vi "Simple_Frequency_Reader.vi"() -> ()   [LabVIEW 2013]
uses:
  <vilib>/S3DK/PMU Recorder Light/PMU Recorder Light.lvlib
panel:
  in  "Quit":bool
  out "Waveform Chart":waveform(sgl)[](graph)
  in  "Refresh Rate":i64(ring)=200 items=["50 Hz"=20, "20 Hz"=50, "10 Hz"=100, "5 Hz"=200, "2 Hz"=500, "1 Hz"=1000, "Every 2 sec"=2000, "Every 5 sec"=5000, "Every 10 sec"=10000, "Every minute"=60000]
  in  "error in (no error)":errorcluster
  out "error out":errorcluster
  # "INPUT"
  # "INTERMEDIATE"
  # "OUTPUT"
  # "USAGE:  Press play. The VI will start the PRL itself and wait for the connection to be established.\n(you will still need to configure the PRL first. If the Simple Frequency Reader works, then this works)"
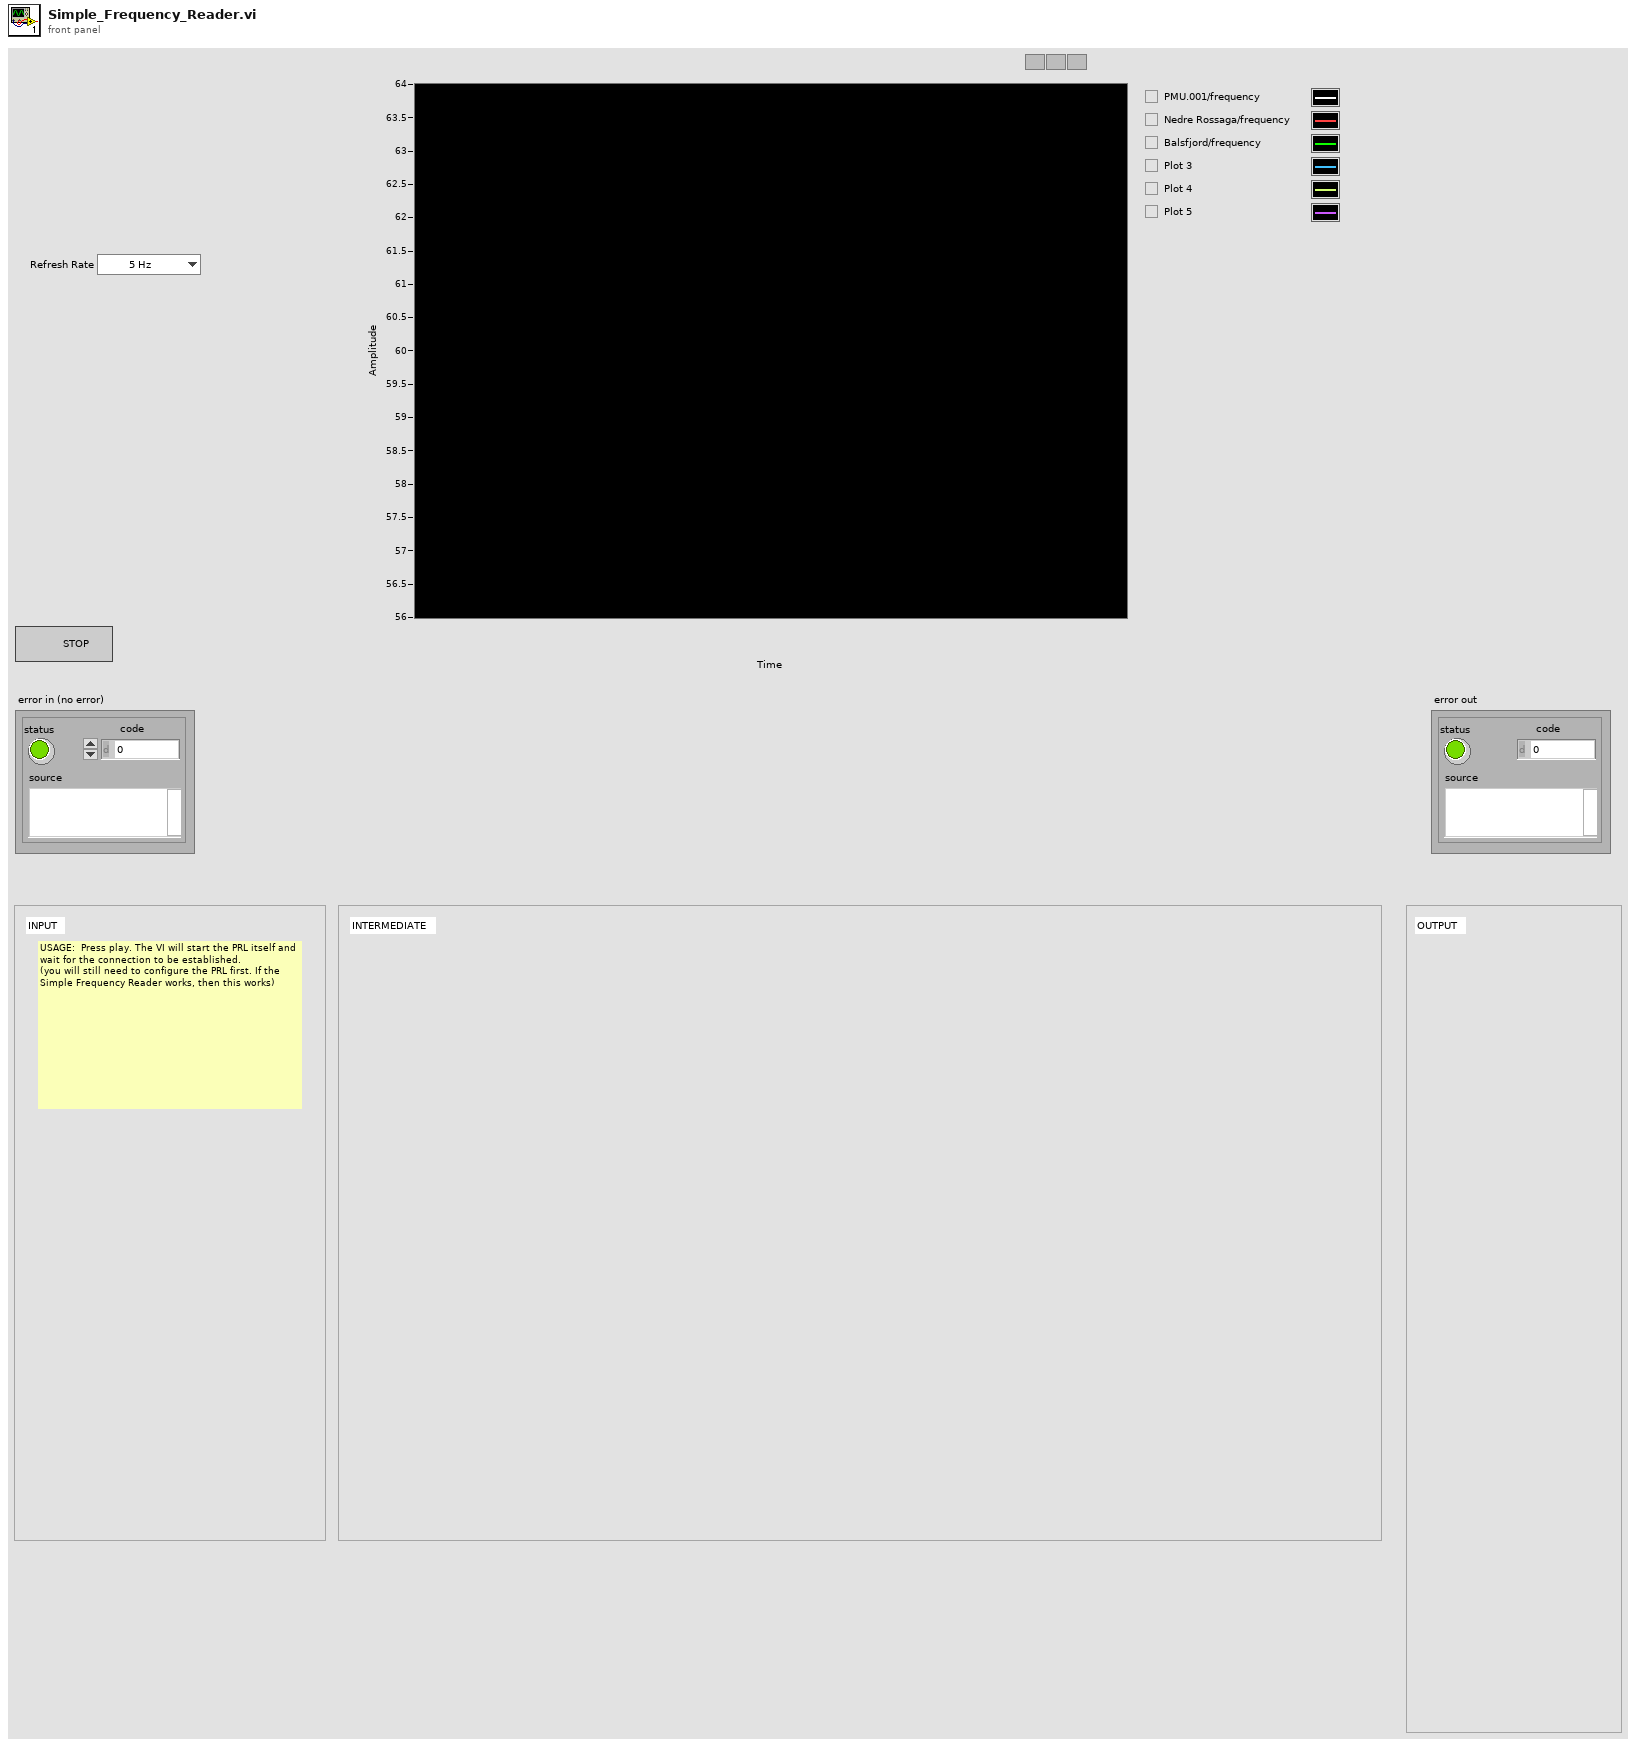
[diagram p1: front panel]
types:
  T1 = enum16{"Run", "Startup", "Get Status", "Pause", "Continue", "Shutdown", "Abort", "Open Panel", "Close Panel"}
  T2 = enum16{"Filter Signals", "Get All Signal Names", "Select Signals on Name", "Select Frequency Only", "Get Selected Signal Names"}
  T3 = cluster{"Phasor":string[], "Analog":string[], "Digital":string[]}
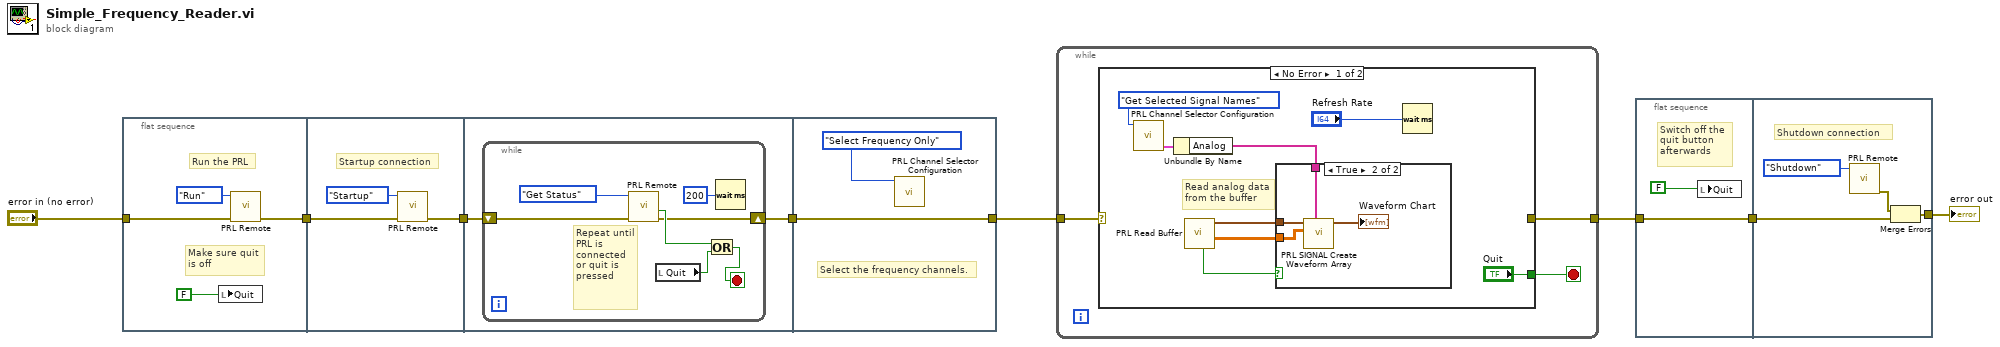
[diagram p0: block diagram]
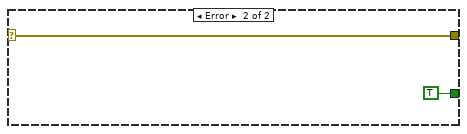
[diagram p3: hidden frame]
diagram:
  n1 = flat-sequence {
    tunnel: "error in (no error)" -> [w10]
    tunnel: [w9] -> w8
    tunnel: w8 -> [w14]
    tunnel: [w13] -> w7
    tunnel: w7 -> [w17]
    tunnel: [w16] -> w6
    tunnel: w6 -> [w25]
    tunnel: [w25] -> w2
    frame #0 {
      # "Make sure quit\nis off"
      # "Run the PRL"
      n2 = local write "Quit"(FALSE ("Quit")) -> ()
      n3 = call <vilib>:"PRL Remote.vi"("error in (no error)"=w10, "Action"=T1."Run") -> ("error out"=w9:errorcluster)  [unwired: 4 in, 5 out]
    }
    frame #1 {
      # "Startup connection"
      n4 = call <vilib>:"PRL Remote.vi"("error in (no error)"=w14, "Action"=T1."Startup") -> ("error out"=w13:errorcluster)  [unwired: 4 in, 5 out]
    }
    frame #2 {
      n5 = while {
        shift-right: [w18] -> w16
        shift-left: w17 -> [w19]
        stop <- w22 stop-if-true
        # "Repeat until PRL is connected or quit is pressed"
        n6 = call <vilib>:"PRL Remote.vi"("error in (no error)"=w19, "Action"=T1."Get Status") -> ("error out"=w18:errorcluster, "Connected"=w20:bool)  [unwired: 4 in, 4 out]
        n7 = local read "Quit"() -> (w21:bool)
        n8 = Or(x=w20, y=w21) -> (x .or. y?=w22:bool)
        n9 = Wait (ms)(milliseconds to wait=u32 200) -> ()  [unwired: 1 out]
      }
    }
    frame #3 {
      # "Select the frequency channels."
      n10 = call <vilib>:"PRL Channel Selector Configuration.vi"("Action"=T2."Select Frequency Only") -> ()  [unwired: 10 in, 1 out]
    }
  }
  n11 = while {
    tunnel: w2 -> [w28]
    tunnel: [w27] -> w3
    stop <- w29 stop-if-true
    n12 = case shown="No Error" w28 {
      selector: w28 -> [_ w43]
      tunnel: ["Quit" TRUE] -> w29
      tunnel: [_ w43] -> w27
      frame No Error {
        # "Read analog data\nfrom the buffer"
        n13 = call <vilib>:"PRL Channel Selector Configuration.vi"("Action"=T2."Get Selected Signal Names") -> ("Signal Names Out"=w35:T3)  [unwired: 10 in]
        n14 = Unbundle By Name(w35) -> ("Analog"=w34:string[])
        n15 = call <vilib>:"PRL Read Buffer .vi"() -> ("Analog Signals"=w31:sgl[][], "Timestamp"=w32:timestamp[], "Has Data"=w33:bool)  [unwired: 6 in, 3 out]
        n16 = case shown="True" w33 {
          tunnel: w32 -> [_ w40]
          tunnel: w31 -> [_ w39]
          tunnel: w34 -> [_ w41]
          frame False {
            # "If there is no new data there is no point in sending them to the plot."
          }
          frame True {
            n17 = call <vilib>:"PRL SIGNAL Create Waveform Array.vi"("Signal Names"=w41, "Analog Signals"=w39, "Timestamp"=w40) -> ("Waveform Array"=→"Waveform Chart":waveform(sgl)[])  [unwired: 8 in]
          }
        }
        n18 = Wait (ms)(milliseconds to wait="Refresh Rate") -> ()  [unwired: 1 out]
      }
      frame Error {
      }
    }
  }
  n19 = flat-sequence {
    tunnel: [w45] -> w5
    tunnel: w3 -> [w45]
    tunnel: w5 -> [w47]
    tunnel: [w46] -> w4
    frame #0 {
      # "Switch off the\nquit button\nafterwards"
      n20 = local write "Quit"(FALSE ("Quit")) -> ()
    }
    frame #1 {
      # "Shutdown connection"
      n21 = call <vilib>:"PRL Remote.vi"("Action"=T1."Shutdown") -> ("error out"=w48:errorcluster)  [unwired: 5 in, 5 out]
      n22 = Merge Errors(w48, w47) -> (w46:errorcluster)
    }
  }
  "error out" <- w4
